vi "Time Filter.vi"(6 "Filter Mode":T1=enum."Include", 8 "error in (no error)":errorcluster, 9 "Filter Time End":timestamp, 10 "Filter Time Start":timestamp, 11 "TDMS Paths In":path[](array[path])) -> (0 "error out":errorcluster, 3 "TDMS Paths Out":path[](array[path]))   [LabVIEW 2017, in "XTree.xctl"]
doc: "Removes files which do not pass the specified time filter."
uses:
  <vilib>/addons/_NIFileIO/XTree/XTree.xctl
  <vilib>/addons/_NIFileIO/XTree/Controls/Filter Mode.ctl
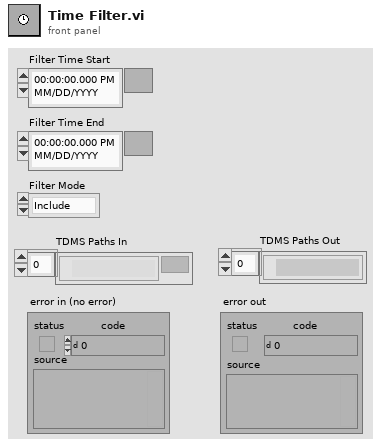
[diagram p1: front panel]
types:
  T1 = typedef "XTree.xctl/Filter Mode.ctl" = enum16{"Exclude", "Include"}
  T2 = enum16{"open", "open or create", "create or replace", "create", "open (read-only)"}
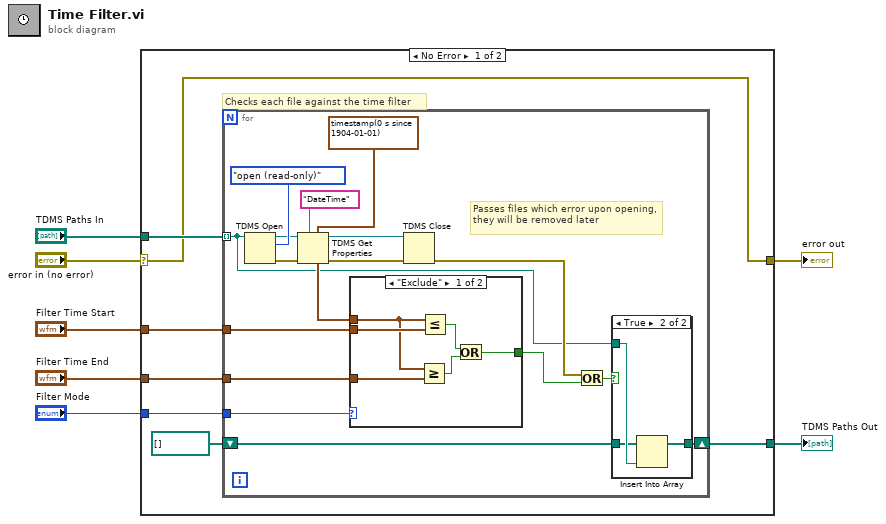
[diagram p0: block diagram]
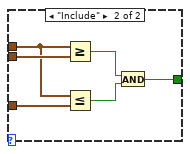
[diagram p3: hidden frame]
diagram:
  n1 = case shown="No Error" "error in (no error)" {
    selector: "error in (no error)" -> [w8 w49]
    tunnel: "TDMS Paths In" -> [w14 w48]
    tunnel: "Filter Mode" -> [w13 _]
    tunnel: "Filter Time Start" -> [w12 _]
    tunnel: "Filter Time End" -> [w11 _]
    tunnel: [w9 w48] -> w3
    tunnel: [w8 w49] -> w2
    frame No Error {
      # "Checks each file against the time filter"
      n2 = for {
        tunnel: w14 -> [w15] mode=indexing
        tunnel: w13 -> [w26]
        tunnel: w12 -> [w24]
        tunnel: w11 -> [w23]
        shift-right: [w19] -> w9
        shift-left: path[] [] -> [w20]
        # "Passes files which error upon opening, they will be removed later"
        n3 = TDMS Open(10:T2."open (read-only)" ("operation (0:open)"), 11:w15) -> (0:w29:errorcluster, 3:w30:refnum<k34>)  [unwired: 5 in]
        n4 = TDMS Get Properties(5:timestamp(0 s since 1904-01-01), 7:"DateTime" ("property name"), 8:w29, 11:w30) -> (0:w21:errorcluster, 3:w22:refnum<k34>, 4:w25:timestamp)  [unwired: 2 in, 3 out]
        n5 = case shown="\"Exclude\"" w26 {
          tunnel: w25 -> [w40 w46]
          tunnel: w24 -> [w41 w47]
          tunnel: w23 -> [w39 w45]
          tunnel: [w36 w42] -> w17
          frame "Exclude" {
            n6 = Greater Or Equal?(x=w40, y=w39) -> (x >= y?=w37:bool)
            n7 = Less Or Equal?(x=w40, y=w41) -> (x <= y?=w38:bool)
            n8 = Or(x=w38, y=w37) -> (x .or. y?=w36:bool)
          }
          frame "Include" {
            n9 = Greater Or Equal?(x=w46, y=w47) -> (x >= y?=w43:bool)
            n10 = Less Or Equal?(x=w46, y=w45) -> (x <= y?=w44:bool)
            n11 = And(x=w43, y=w44) -> (x .and. y?=w42:bool)
          }
        }
        n12 = TDMS Close(8:w21, 11:w22) -> (0:w16:errorcluster)  [unwired: 1 out]
        n13 = Or(x=w16, y=w17) -> (x .or. y?=w18:bool)
        n14 = case shown="True" w18 {
          tunnel: w20 -> [w32 w33]
          tunnel: w15 -> [_ w35]
          tunnel: [w32 w34] -> w19
          frame False {
          }
          frame True {
            n15 = Insert Into Array(array=w33, new element=w35) -> (w34:path[])  [unwired: 1 in]
          }
        }
      }
    }
    frame Error {
    }
  }
  "TDMS Paths Out" <- w3
  "error out" <- w2
